vi "FdxCmdTxEDECreatePortCvi.vi"(8 "error in":errorcluster, 9 "EDETxDescription":T1={"EDESourceId"=1, "EDESubscriberHandle"=0}, 10 "EDEUdpDescription":T2={"PortType"=enum."FDX_UDP_QUEUEING", "UdpSrc"=2000, "IpSrc"=167846145, "VlId"=60, "IpDst"=3772776508, "UdpDst"=2000, "SubVlId"=1, "UdpNumBufMessages"=10, "UdpMaxMessageSize"=64, "UdpSamplingRate"=0}, 11 "InstrumentHandle":u32) -> (0 "error out":errorcluster, 2 "EDEHandle":u32, 3 "InstrumentHandle":u32)   [LabVIEW 2020, in "AIM664LV.lvlib"]
doc: "This function is used to create and configure a new EDE enabled UDP port. Default settings after creation of the EDE port are:\n- UDP port enabled\n- Error injection: OFF\n- Skew (redundant mode only): 0 usec.\nTo change the settings of the UDP port the function FdxCmdTxUDPControl can be used. This function can be used only if transmitter is not running."
uses:
  AIM664LV.lvlib
  AFDX_LibraryAdmin/FdxGlobalDllPath.vi
panel:
  # "Inputs"
  # "Outputs"
  # "Hex"
  # "Hex"
  # "Hex"
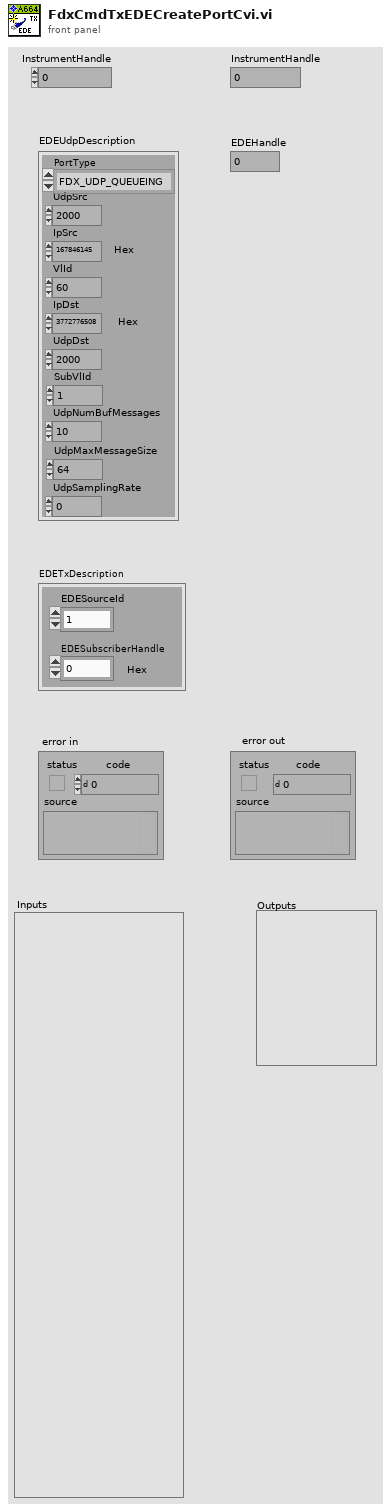
[diagram p1: front panel]
types:
  T1 = cluster{"EDESourceId":u32, "EDESubscriberHandle":u32}
  T2 = cluster{"PortType":enum32{"FDX_UDP_SAMPLING", "FDX_UDP_QUEUEING"}, "UdpSrc":u32, "IpSrc":u32, "VlId":u32, "IpDst":u32, "UdpDst":u32, "SubVlId":u32, "UdpNumBufMessages":u32, "UdpMaxMessageSize":u32, "UdpSamplingRate":u32}
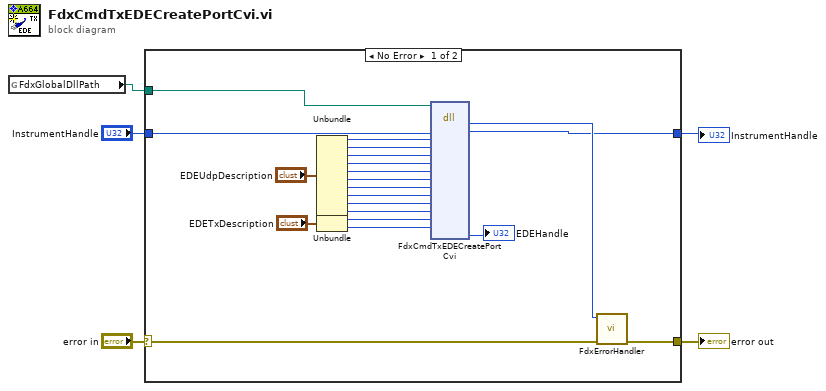
[diagram p0: block diagram]
diagram:
  n1 = global read "FdxGlobalDllPath.vi" "FdxGlobalDllPath"() -> (w3:path)
  n2 = case shown="No Error" "error in" {
    selector: "error in" -> [w25 w28]
    tunnel: [w26 w28] -> w5
    tunnel: w3 -> [w8 _]
    tunnel: "InstrumentHandle" -> [w7 w27]
    tunnel: [w6 w27] -> w1
    frame No Error {
      n3 = Unbundle("EDEUdpDescription") -> ("PortType"=w22:enum32{"FDX_UDP_SAMPLING", "FDX_UDP_QUEUEING"}, "UdpSrc"=w21:u32, "IpSrc"=w20:u32, "VlId"=w19:u32, "IpDst"=w18:u32, "UdpDst"=w17:u32, "SubVlId"=w14:u32, "UdpNumBufMessages"=w13:u32, "UdpMaxMessageSize"=w12:u32, "UdpSamplingRate"=w11:u32)
      n4 = Unbundle("EDETxDescription") -> ("EDESourceId"=w10:u32, "EDESubscriberHandle"=w9:u32)
      n5 = dll-call lib="aim_fdx.19.dll" fn="FdxCmdTxEDECreatePortCvi"(path in=w8, "InstrumentHandle"=w7, "PortType"=w22, "UdpSrc"=w21, "IpSrc"=w20, "VlId"=w19, "IpDst"=w18, "UdpDst"=w17, "SubVlId"=w14, "UdpNumBufMessages"=w13, "UdpMaxMessageSize"=w12, "UdpSamplingRate"=w11, "EDESourceId"=w10, "EDESubscriberHandle"=w9) -> ("status"=w24:i32, "InstrumentHandle"=w6:u32, "EDEHandle"=→"EDEHandle":u32)  [unwired: 13 in, 4 out]
      n6 = call "FdxErrorHandler.vi"("error in"=w25, "AIM Error"=w24) -> ("error out"=w26:errorcluster)  [unwired: 9 in]
    }
    frame Error {
    }
  }
  "error out" <- w5
  "InstrumentHandle" <- w1
